vi "Initialize Bus Monitor.vi"(8 "error in":errorcluster, 11 "module handle":u32) -> (0 "error out":errorcluster, 3 "module handle out":u32)   [LabVIEW 2020, in "AIM MIL-STD-1553 Hardware API.lvlib"]
uses:
  AIM MIL-STD-1553 Hardware API.lvlib
  Global - Disable Hardware API Constant.vi
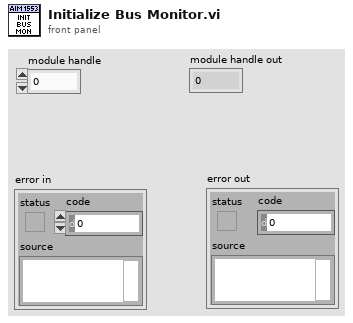
[diagram p1: front panel]
types:
  T1 = enum16{"Enabled (Default)", "Disabled for Unit Testing"}
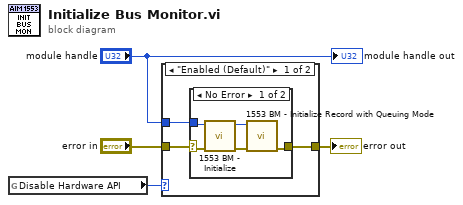
[diagram p0: block diagram]
diagram:
  n1 = global read "Global - Disable Hardware API Constant.vi" "Disable Hardware API"() -> (w4:T1)
  n2 = case shown="\"Enabled (Default)\"" w4 {
    tunnel: "error in" -> [w7 w14]
    tunnel: [w6 w14] -> w2
    tunnel: "module handle" -> [w5 _]
    frame "Enabled (Default)" {
      n3 = case shown="No Error" w7 {
        selector: w7 -> [w9 w13]
        tunnel: [w10 w13] -> w6
        tunnel: w5 -> [w8 _]
        frame No Error {
          n4 = call <instrlib>:"1553 BM - Initialize.vi"("Error In (none)"=w9, "Module Handle"=w8) -> ("Error Out"=w12:errorcluster, "Module Handle out"=w11:u32)  [unwired: 8 in]
          n5 = call <instrlib>:"1553 BM - Initialize Record with Queuing Mode.vi"("Error In (none)"=w12, "Module Handle"=w11) -> ("Error Out"=w10:errorcluster)  [unwired: 8 in, 1 out]
        }
        frame Error {
        }
      }
    }
    frame "Disabled for Unit Testing" {
    }
  }
  "error out" <- w2
  "module handle out" <- "module handle"
